vi "CheckForErrors.vi"(8 "error in (no error)":errorcluster, 11 "STOMP in":refnum<class "STOMP.lvclass">) -> (0 "error out":errorcluster, 2 "stomp error msg":errorcluster, 3 "STOMP out":refnum<class "STOMP.lvclass">)   [LabVIEW 2017, in "LabVIEW STOMP.lvlib" / "STOMP.lvclass"]
uses:
  STOMP.lvclass
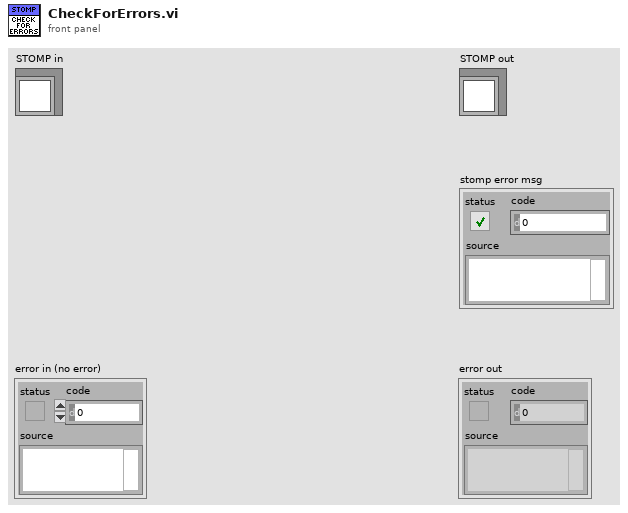
[diagram p1: front panel]
types:
  T1 = typedef "STOMP Connection Manager.lvclass/ObjectAttributes.ctl" = cluster{"address":string, "port":u16, "ConnectionRef":refnum<k5>, "messageQueue":refnum<queue>, "receiptQueue":refnum<queue>, "errorQueue":refnum<queue>, "sendQueue":refnum<queue>, "currentReceiptNumber":u64, "currentSubscriptionId":u64, "closeConnection":bool, "activeSubscriptions":T2[]}
  T2 = typedef "LabVIEW STOMP.lvlib/STOMP.lvclass/Type_ActiveSubscription.ctl" = cluster{"id":u64, "receipt":bool, "Destination":string, "ack":T3, "headers":T4[]}
  T3 = typedef "LabVIEW STOMP.lvlib/STOMP.lvclass/Type_AckHeader.ctl" = enum16{"auto", "client", "client-individual"}
  T4 = typedef "LabVIEW STOMP.lvlib/STOMP.lvclass/Type_FrameHeader.ctl" = cluster{"Header":string, "Value":string}
  T5 = typedef "LabVIEW STOMP.lvlib/STOMP.lvclass/Type_ServerFrame.ctl" = cluster{"Type":T6, "Headers":cluster{"Header":string, "Value":string}[], "Body":string}
  T6 = typedef "LabVIEW STOMP.lvlib/STOMP.lvclass/Type_ServerFrameType.ctl" = enum16{"Undefined", "MESSAGE", "CONNECTED", "RECEIPT", "ERROR"}
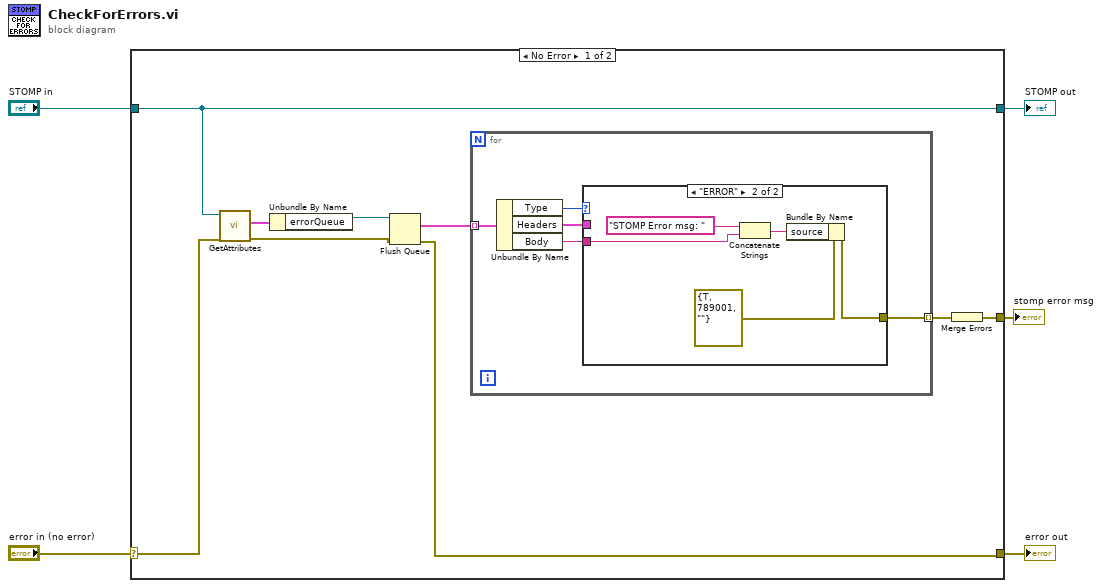
[diagram p0: block diagram]
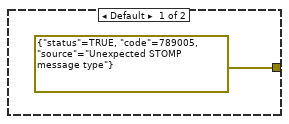
[diagram p2: hidden frame]
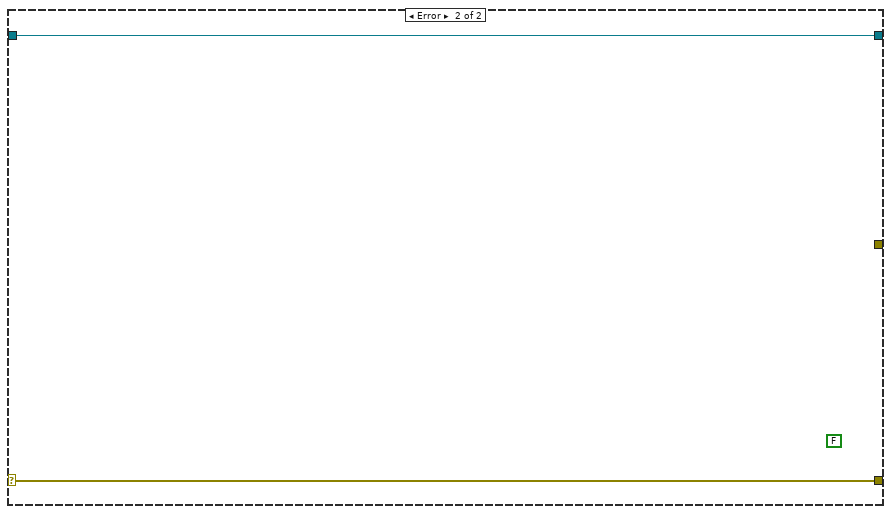
[diagram p3: hidden frame]
diagram:
  n1 = case shown="No Error" "error in (no error)" {
    selector: "error in (no error)" -> [w11 w27]
    tunnel: [w9 w27] -> w4
    tunnel: [w13 w26] -> w2
    tunnel: "STOMP in" -> [w13 w26]
    tunnel: [w6 _] -> w1
    frame No Error {
      n2 = call-dynamic "GetAttributes.vi"("error in (no error)"=w11, "STOMP in"=w13) -> ("error out"=w7:errorcluster, "attributes"=w12:T1)  [unwired: 7 in, 1 out]
      n3 = Unbundle By Name(w12) -> ("errorQueue"=w14:refnum<queue>)
      n4 = Flush Queue(queue=w14, error in (no error)=w7) -> (remaining elements=w8:T5[], error out=w9:errorcluster)  [unwired: 1 out]
      n5 = for {
        tunnel: [w19] -> w10 mode=indexing
        tunnel: w8 -> [w15] mode=indexing
        n6 = Unbundle By Name(w15) -> ("Type"=w18:T6, "Headers"=w17:cluster{"Header":string, "Value":string}[], "Body"=w16:string)
        n7 = case shown="\"ERROR\"" w18 {
          tunnel: w17 -> [_ _]
          tunnel: w16 -> [_ w24]
          tunnel: [errorcluster {"status"=TRUE, "code"=789005, "source"="Unexpected STOMP message type"} ("error constant") w21] -> w19
          frame Default {
          }
          frame "ERROR" {
            n8 = Concatenate Strings("STOMP Error msg: ", w24) -> (w22:string)
            n9 = Bundle By Name(cluster=errorcluster {"status"=TRUE, "code"=789001, "source"=""} ("error constant"), "source"=w22) -> (w21:errorcluster)
          }
        }
      }
      n10 = Merge Errors(w10) -> (w6:errorcluster)
    }
    frame Error {
      (unwired) FALSE ("timed out?")
    }
  }
  "error out" <- w4
  "STOMP out" <- w2
  "stomp error msg" <- w1
